vi "Write Data.vi"(8 "error in (no error)":errorcluster, 9 "Publication Time":timestamp, 10 "Value":variant, 11 "NotifierTransport In":refnum<class "NotifierTransport.lvclass">) -> (0 "error out":errorcluster, 3 "NotifierTransport Out":refnum<class "NotifierTransport.lvclass">)   [LabVIEW 2018, in "MVA Framework.lvlib" / "NotifierTransport.lvclass"]
doc: "写入数据"
uses:
  NotifierTransport.lvclass
  <vilib>/ErrorRing/Error Ring.xnode
  <vilib>/Utility/error.llb/Error Cluster From Error Code.vi
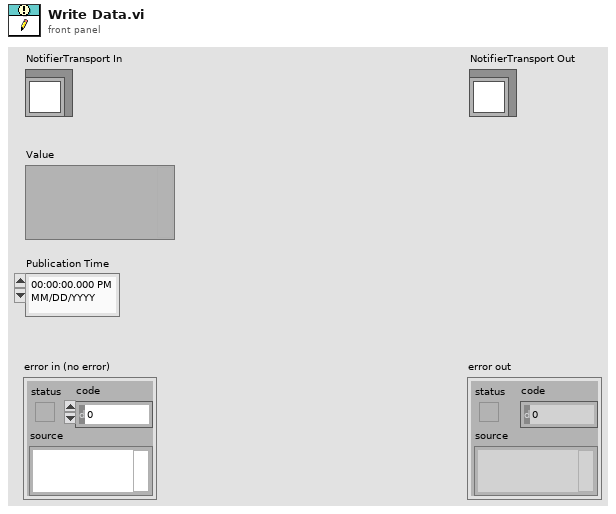
[diagram p1: front panel]
types:
  T1 = cluster{"Value":variant, "Publication Time":timestamp}
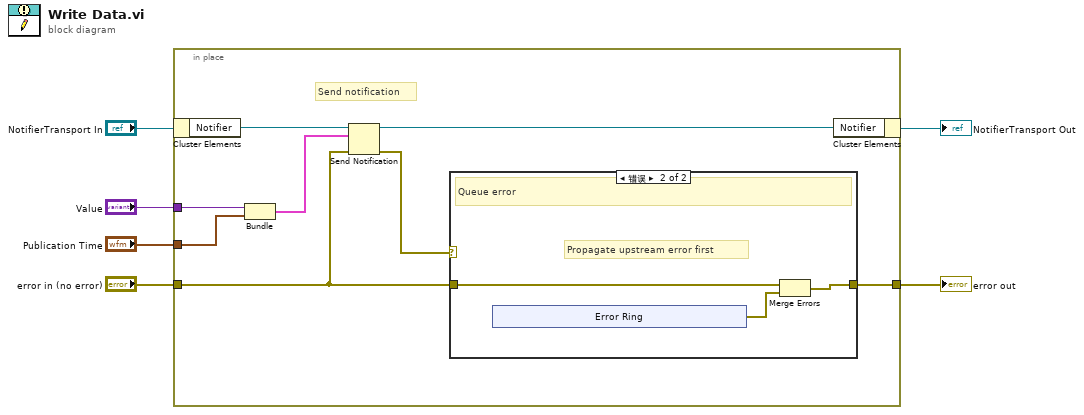
[diagram p0: block diagram]
diagram:
  n1 = in-place {
    in-place-border: "error in (no error)" -> [w8]
    in-place-border: "Value" -> [w14]
    in-place-border: "Publication Time" -> [w13]
    in-place-border: [w9] -> w3
    # "Send notification"
    n2 = in-place-cluster #1("NotifierTransport In") -> ("Notifier"=w11:refnum<notifier>)
    n3 = Bundle("Value"=w14, "Publication Time"=w13) -> (w12:T1)  [unwired: 1 in]
    n4 = Send Notification(notification=w12, notifier=w11, error in (no error)=w8) -> (notifier out=w10:refnum<notifier>, error out=w7:errorcluster)
    n5 = case shown="错误" w7 {
      selector: w7 -> [w15 _]
      tunnel: [w15 w18] -> w9
      tunnel: w8 -> [_ w16]
      frame No Error {
        # "Things seem normal"
      }
      frame Error {
        # "Propagate upstream error first"
        # "Queue error"
        n6 = xnode "Error Ring"() -> ("错误输出"=w17:errorcluster)
        n7 = Merge Errors(w16, w17) -> (w18:errorcluster)
      }
    }
    n8 = in-place-cluster #1("Notifier"=w10) -> (→"NotifierTransport Out":refnum<class "NotifierTransport.lvclass">)
  }
  "error out" <- w3
